vi "ConfigInputChangeReagent.vi"(1 "MulticolumnListbox in":refnum<vi>, 3 "ItemNames in":string[][](array[string])) -> (0 "ItemNames out":string[][](array[string]))   [LabVIEW 2018, in "Config.lvlib"]
uses:
  Config.lvlib
panel:
  in  "Reagent Nr.":u8(ring)=1 items=["All", "1", "2", "3", "4", "5", "6", "7", "8"]
  in  "Replace":bool
  in  "Insert":bool
  in  "Append":bool
  in  "Flushing Time":dbl=1.0 min=1.0 step=1.0 format="%<%H:%M:%S>t"
  # "Flush Step"
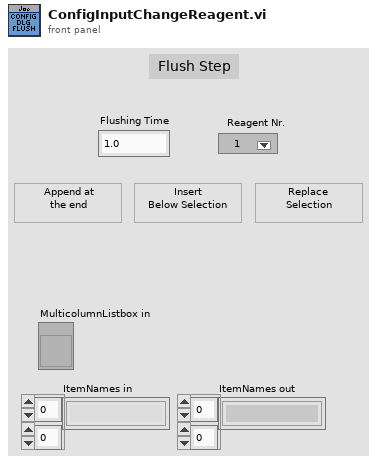
[diagram p1: front panel]
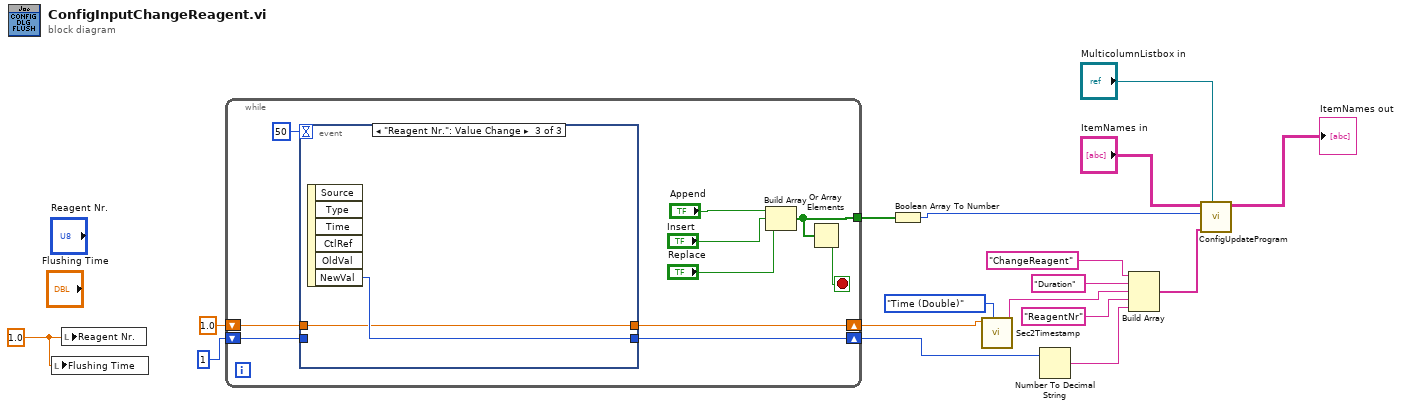
[diagram p0: block diagram]
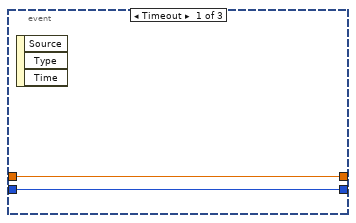
[diagram p2: hidden frame]
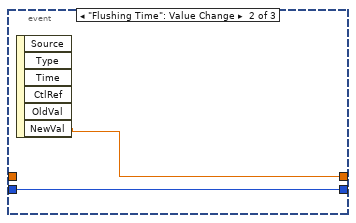
[diagram p3: hidden frame]
diagram:
  w17 = 1.0 ("Mixing Cycles")
  n1 = local write "Flushing Time"(w17) -> ()
  n2 = local write "Reagent Nr."(w17) -> ()
  n3 = while {
    tunnel: [w22] -> w16
    shift-right: [w21] -> w1
    shift-left: 1.0 ("NewVal") -> [w20]
    shift-right: [w19] -> w2
    shift-left: u8 1 -> [w18]
    stop <- w23 stop-if-true
    n4 = event shown="[2] \"Reagent Nr.\": Value Change" {
      selector: _ -> [_ _ _]
      dyn-events: _ -> [_ _ _]
      timeout: 50 -> [_ _ _]
      tunnel: [w29 w31 w32] -> w21
      tunnel: w20 -> [w29 _ w32]
      tunnel: [w28 w30 w33] -> w19
      tunnel: w18 -> [w28 w30 _]
      event Timeout {
        n5 = event-data() -> ()  [unwired: 1 in, 3 out]
      }
      event "Flushing Time": Value Change {
        n6 = event-data() -> ("NewVal"=w31:dbl)  [unwired: 1 in, 5 out]
      }
      event "Reagent Nr.": Value Change {
        n7 = event-data() -> ("NewVal"=w33:u8)  [unwired: 1 in, 5 out]
      }
    }
    n8 = Build Array("Append", "Insert", "Replace") -> (w22:bool[])
    n9 = Or Array Elements(Boolean array=w22) -> (logical OR=w23:bool)
  }
  n10 = Boolean Array To Number(Boolean array=w16) -> (number=w14:u32)
  n11 = call "Sec2Timestamp.vi"("Input Selection"=enum32{"Time (Double)", "Time (Time Stamp)"}."Time (Double)", "Input Time (Double)"=w1) -> ("time string"=w4:string)  [unwired: 7 in, 2 out]
  n12 = Number To Decimal String(number=w2) -> (decimal integer string=w6:string)  [unwired: 1 in]
  n13 = Build Array("ChangeReagent", "Duration", w4, "ReagentNr", w6) -> (w3:string[])
  n14 = call "ConfigUpdateProgram.vi"("MulticolumnListbox in"="MulticolumnListbox in", "New Element"=w3, "Operation"=w14, "ItemNames in"="ItemNames in") -> ("ItemNames out"=→"ItemNames out":string[][])  [unwired: 7 in]
